vi "account manager.vi"(8 "error in":errorcluster, 10 "Users":T1[](array[typedef]), 11 "action":string="Init") -> (0 "error out":errorcluster, 3 "Users":T1[](array[typedef]))   [LabVIEW 2015]
uses:
  User data.ctl
  <vilib>/Utility/file.llb/Write Delimited Spreadsheet (string).vi
  <vilib>/Utility/file.llb/Read Delimited Spreadsheet (string).vi
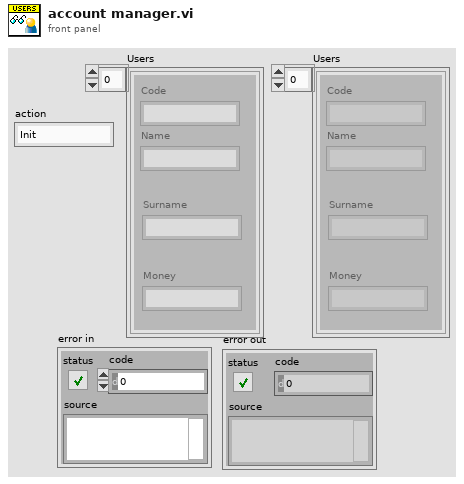
[diagram p1: front panel]
types:
  T1 = typedef "User data.ctl" = cluster{"Code":string, "Name":string, "Surname":string, "Money":string}
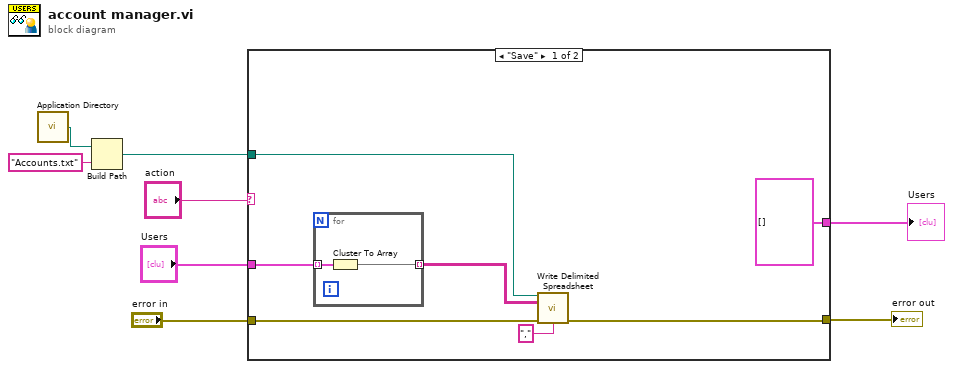
[diagram p0: block diagram]
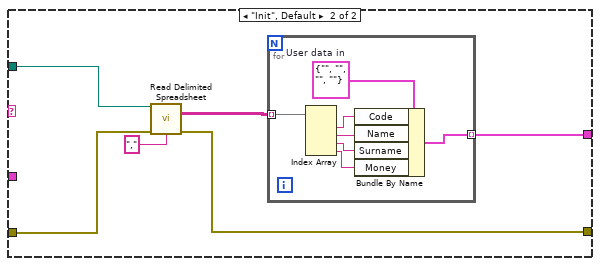
[diagram p2: hidden frame]
diagram:
  n1 = call <vilib>:"Application Directory.vi"() -> ("Application Directory"=w6:path)
  n2 = Build Path(base path=w6, name or relative path="Accounts.txt") -> (appended path=w8:path)
  n3 = case shown="\"Save\"" "action" {
    tunnel: w8 -> [w10 w23]
    tunnel: [T1[] [] w21] -> w5
    tunnel: [w12 w19] -> w3
    tunnel: "error in" -> [w13 w18]
    tunnel: "Users" -> [w14 _]
    frame "Save" {
      n4 = for {
        tunnel: w14 -> [w17] mode=indexing
        tunnel: [w16] -> w11 mode=indexing
        n5 = Cluster To Array(cluster=w17) -> (array=w16:string[])
      }
      n6 = call-poly <vilib>:"Write Delimited Spreadsheet.vi"("file path (dialog if empty)"=w10, "2D data"=w11, "error in (no error)"=w13, "delimiter (\\t)"="," ("delimiter (\\t)")) -> ("error out"=w12:errorcluster)  [unwired: 10 in, 1 out]
    }
    frame "Init", Default {
      n7 = call-poly <vilib>:"Read Delimited Spreadsheet.vi"("file path (dialog if empty)"=w23, "error in (no error)"=w18, "delimiter (\\t)"="," ("delimiter (\\t)")) -> ("all rows"=w20:string[][], "error out"=w19:errorcluster)  [unwired: 7 in, 4 out]
      n8 = for {
        tunnel: w20 -> [w30] mode=indexing
        tunnel: [w25] -> w21 mode=indexing
        w29 = T1 {"Code"="", "Name"="", "Surname"="", "Money"=""}  # User data in
        n9 = Index Array(array=w30) -> (element #1=w28:string, element #2=w27:string, element #3=w26:string, element #4=w24:string)  [unwired: 4 in]
        n10 = Bundle By Name(cluster=w29, "Code"=w28, "Name"=w27, "Surname"=w26, "Money"=w24) -> (w25:T1)
      }
    }
  }
  "Users" <- w5
  "error out" <- w3
